vi "GBL DataQ Ref.vi"() -> ()   [LabVIEW 2019]
doc: "Developed by Kevin Thompson\nkevin@thompsonengineering.net\n\nCopyright 2018-2020\nThompson Engineering, LLC"
panel:
  in  "ProcData DataQ xRef":u32
  in  "LogMeas DataQ xRef":u32
  in  "DAQMeas DataQ xRef":u32
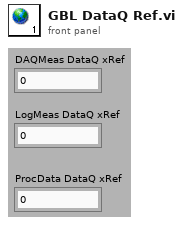
[diagram p1: front panel]
diagram:
